vi "TPNT_CallDevice.vi"(0 "CmdStringIn":string, 11 "error in (no error)":errorcluster) -> (4 "ImmedReplyString":string, 15 "error out":errorcluster)   [LabVIEW 2016]
panel:
  in  "AVAPP Cmd Proc":refnum<vi>
  out "Cmd Option":string
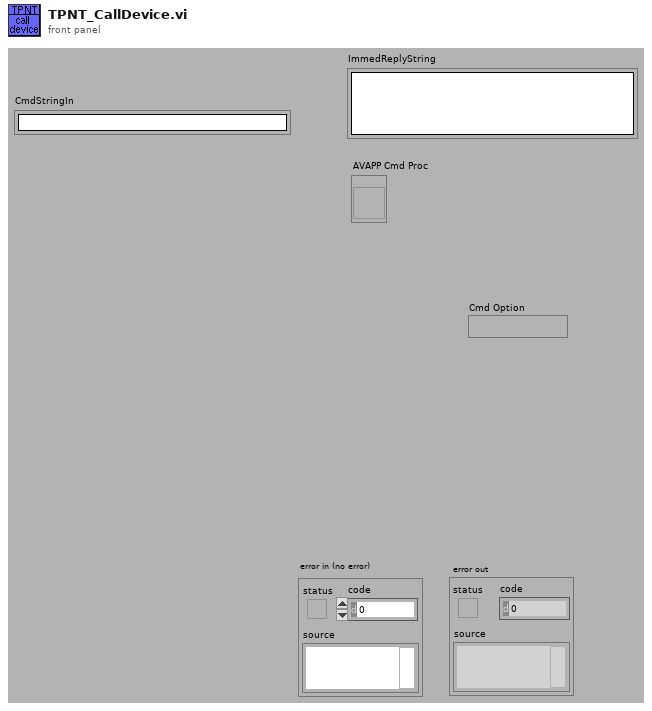
[diagram p1: front panel]
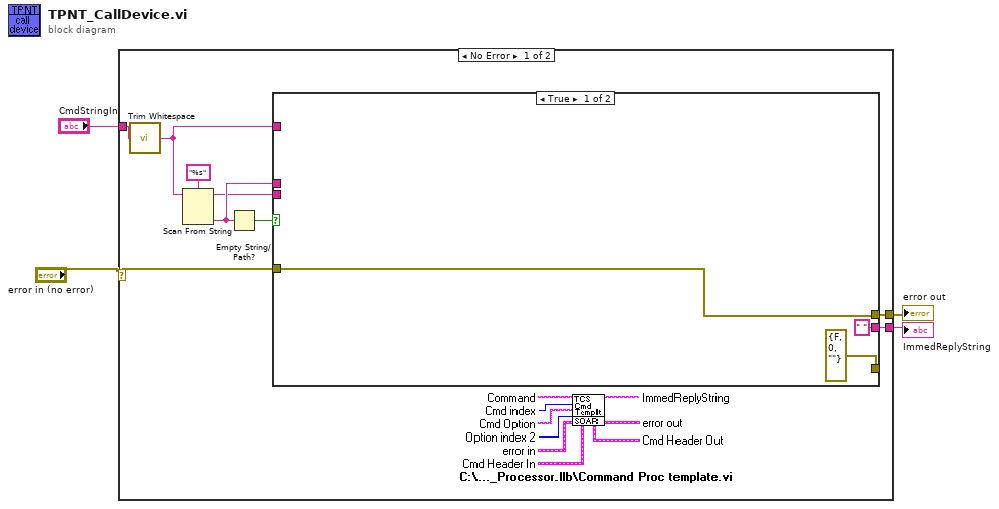
[diagram p0: block diagram]
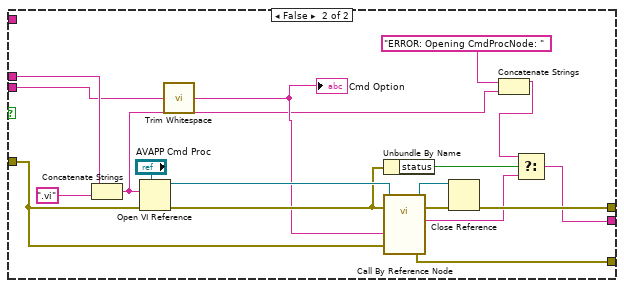
[diagram p2: hidden frame]
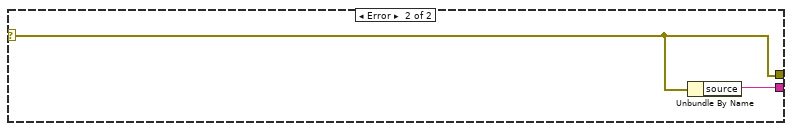
[diagram p3: hidden frame]
diagram:
  n1 = case shown="No Error" "error in (no error)" {
    selector: "error in (no error)" -> [w5 w36]
    tunnel: [w13 w35] -> w4
    tunnel: [w12 w36] -> w3
    tunnel: "CmdStringIn" -> [w11 _]
    frame No Error {
      n2 = call <vilib>:"Trim Whitespace.vi"("string"=w11) -> ("trimmed string"=w10:string)  [unwired: 1 in]
      n3 = Scan From String(format string="%s", input string=w10) -> (remaining string=w6:string, output 1=w7:string)  [unwired: 2 in, 3 out]
      n4 = Empty String/Path?(string/path=w7) -> (empty?=w8:bool)
      n5 = case shown="True" w8 {
        tunnel: [" " w26] -> w13
        tunnel: [w16 w28] -> w12
        tunnel: w5 -> [w16 w17]
        tunnel: [errorcluster {"status"=FALSE, "code"=0, "source"=""} ("error out") w24] -> _
        tunnel: w10 -> [_ _]
        tunnel: w7 -> [_ w23]
        tunnel: w6 -> [_ w22]
        frame True {
        }
        frame False {
          n6 = Concatenate Strings(w23, ".vi" ("Substring")) -> (w19:string)
          n7 = Open VI Reference(type specifier VI Refnum (for type only)="AVAPP Cmd Proc", vi path=w19, error in (no error)=w17) -> (vi reference=w33:refnum<vi>, error out=w27:errorcluster)  [unwired: 3 out]
          n8 = call <vilib>:"Trim Whitespace.vi"("string"=w22) -> ("trimmed string"=w21:string)  [unwired: 1 in]
          "Cmd Option" <- w21
          n9 = Unbundle By Name(w27) -> ("status"=w31:bool)
          n10 = call-by-ref "Call By Reference Node"(reference=w33, error in=w27, "Cmd"=w21, "error in"=w17) -> (reference out=w29:refnum<vi>, error out=w30:errorcluster, "ImmedReplyString"=w25:string, 15:"error out"=w24:errorcluster)  [unwired: 12 in]
          n11 = Close Reference(reference=w29, error in (no error)=w30) -> (error out=w28:errorcluster)
          n12 = Concatenate Strings("ERROR: Opening CmdProcNode: " ("t"), w19) -> (w18:string)
          n13 = Select(t=w18, s=w31, f=w25) -> (s? t:f=w26:string)
        }
      }
    }
    frame Error {
      n14 = Unbundle By Name(w36) -> ("source"=w35:string)
    }
  }
  "ImmedReplyString" <- w4
  "error out" <- w3
